vi "Get User.vi"(8 "error IO":errorcluster, 10 "Pointer":i32, 11 "VISA resource name":refnum<visa-resource-name>) -> (0 "error Out":errorcluster, 1 "Password":string, 2 "User Name":string, 3 "VISA resource Out":refnum<visa-resource-name>, 4 "Access Level":u16, 5 "User Found?":bool)   [LabVIEW 2012, in "Associated Research 78XX Series.lvlib"]
uses:
  <instrlib>/Associated Research 78XX Series/Associated Research 78XX Series.lvlib
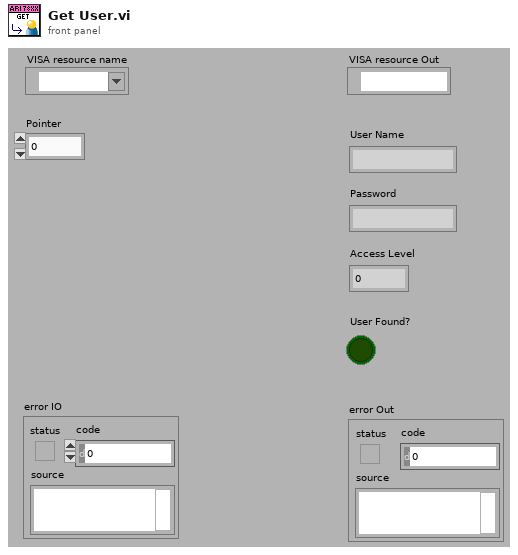
[diagram p1: front panel]
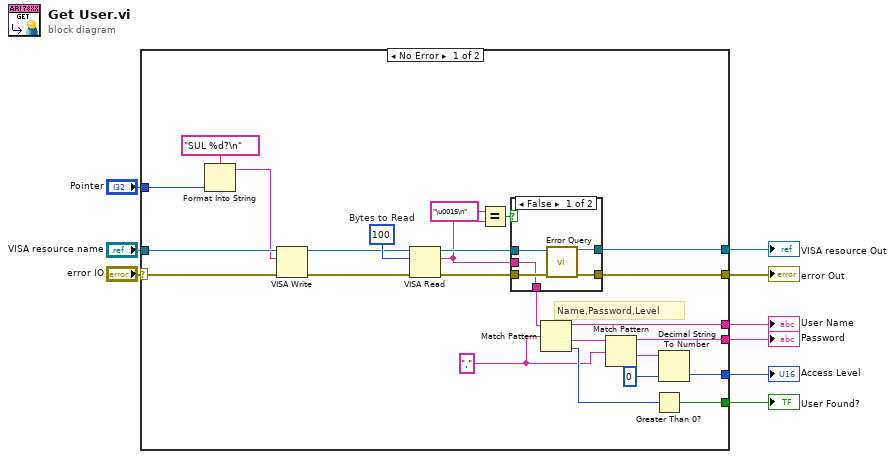
[diagram p0: block diagram]
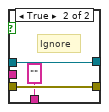
[diagram p2: hidden frame]
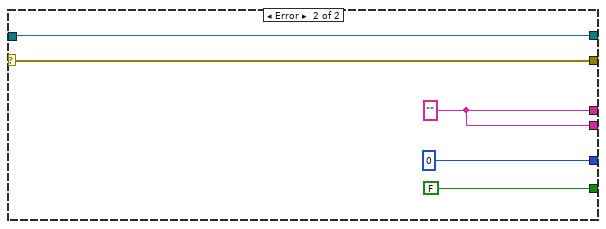
[diagram p3: hidden frame]
diagram:
  n1 = case shown="No Error" "error IO" {
    selector: "error IO" -> [w34 w47]
    tunnel: [w31 w47] -> w6
    tunnel: [w32 w46] -> w7
    tunnel: "VISA resource name" -> [w33 w46]
    tunnel: "Pointer" -> [w13 _]
    tunnel: [w26 w45] -> w4
    tunnel: [w25 w45] -> w3
    tunnel: [w24 u16 0] -> w2
    tunnel: [w23 FALSE] -> w1
    frame No Error {
      w21 = u32 100  # Bytes to Read
      w28 = "," ("regular expression")
      # "Name,Password,Level"
      n2 = Format Into String(format string="SUL %d?\n" ("Command to Send (empty)"), w13) -> (resulting string=w12:string)  [unwired: 2 in, 1 out]
      n3 = VISA Write(VISA resource name=w33, write buffer=w12, error in (no error)=w34) -> (VISA resource name out=w11:refnum<visa-resource-name>, error out=w10:errorcluster)  [unwired: 1 out]
      n4 = VISA Read(VISA resource name=w11, byte count=w21, error in (no error)=w10) -> (VISA resource name out=w20:refnum<visa-resource-name>, read buffer=w18:string, error out=w19:errorcluster)  [unwired: 1 out]
      n5 = Equal?(x="\u0015\n" ("regular expression"), y=w18) -> (x = y?=w16:bool)
      n6 = case shown="False" w16 {
        tunnel: [w39 w41] -> w32
        tunnel: [w38 w42] -> w31
        tunnel: w20 -> [w37 w41]
        tunnel: w19 -> [w36 w42]
        tunnel: w18 -> [w35 _]
        tunnel: [w35 "" ("read buffer")] -> w15
        frame False {
          n7 = call <instrlib>:"Error Query.vi"("VISA resource name"=w37, "error in (no error)"=w36) -> ("VISA resource name out"=w39:refnum<visa-resource-name>, "error out"=w38:errorcluster)  [unwired: 10 in, 2 out]
        }
        frame True {
          # "Ignore"
        }
      }
      n8 = Match Pattern(string=w15, regular expression=w28) -> (before substring=w26:string, after substring=w27:string, offset past match=w30:i32)  [unwired: 1 in, 1 out]
      n9 = Match Pattern(string=w27, regular expression=w28) -> (before substring=w25:string, after substring=w29:string)  [unwired: 1 in, 2 out]
      n10 = Greater Than 0?(x=w30) -> (x > 0?=w23:bool)
      n11 = Decimal String To Number(string=w29, default (0L)=u16 0) -> (number=w24:u16)  [unwired: 1 in, 1 out]
    }
    frame Error {
      w45 = ""
    }
  }
  "VISA resource Out" <- w7
  "error Out" <- w6
  "User Found?" <- w1
  "Password" <- w3
  "Access Level" <- w2
  "User Name" <- w4
